vi "monitor fpga rm window status and set dynamic button state.vi"(8 "error in (no error)":errorcluster) -> (0 "error out":errorcluster)   [LabVIEW 2016, in "FPGA RM System Definition API.lvlib"]
uses:
  FPGA RM System Definition API.lvlib
  <vilib>/NI VeriStand/Custom Device API/Custom Device API.lvlib
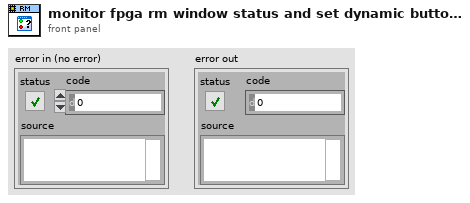
[diagram p1: front panel]
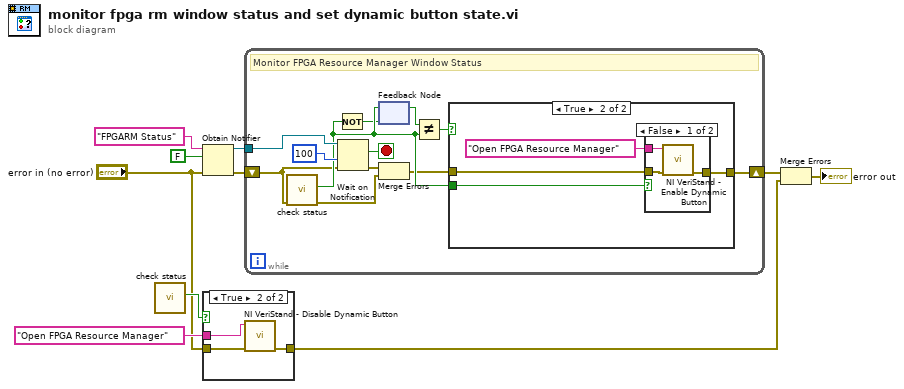
[diagram p0: block diagram]
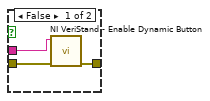
[diagram p2: hidden frame]
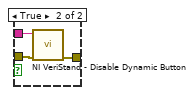
[diagram p4: hidden frame]
diagram:
  n1 = call "check status.vi"() -> ("status"=w6:bool)  [unwired: 10 in, 1 out]
  n2 = Obtain Notifier(name (unnamed)="FPGARM Status", notification data type=FALSE, error in (no error)="error in (no error)") -> (notifier out=w8:refnum<notifier>, error out=w4:errorcluster)  [unwired: 1 in, 1 out]
  n3 = case shown="True" w6 {
    tunnel: "Open FPGA Resource Manager" ("Button ID") -> [w13 w16]
    tunnel: "error in (no error)" -> [w12 w15]
    tunnel: [w11 w14] -> w2
    frame False {
      n4 = call <vilib>:"NI VeriStand - Enable Dynamic Button.vi"("error in (no error)"=w12, "Button ID"=w13) -> ("error out"=w11:errorcluster)  [unwired: 9 in]
    }
    frame True {
      n5 = call <vilib>:"NI VeriStand - Disable Dynamic Button.vi"("error in (no error)"=w15, "Button ID"=w16) -> ("error out"=w14:errorcluster)  [unwired: 9 in]
    }
  }
  n6 = while {
    tunnel: w8 -> [w28]
    shift-right: [w17] -> w3
    shift-left: w4 -> [w21]
    stop <- w27 stop-if-true
    # "Monitor FPGA Resource Manager Window Status"
    n7 = call "check status.vi"("error in (no error)"=w21) -> ("error out"=w19:errorcluster, "status"=w23:bool)  [unwired: 9 in]
    n8 = Not(x=w23) -> (.not. x?=w22:bool)
    n9 = Wait on Notification(notifier=w28, timeout in ms (-1)=100, error in (no error)=w21) -> (notification=w27:bool, error out=w20:errorcluster)  [unwired: 1 in, 2 out]
    n10 = feedback-in #1(w23) -> ()
    n11 = feedback #1(w22) -> (w25:bool)
    n12 = Merge Errors(w20, w19) -> (w18:errorcluster)
    n13 = Not Equal?(x=w25, y=w23) -> (x != y?=w24:bool)
    n14 = case shown="True" w24 {
      tunnel: w23 -> [_ w32]
      tunnel: w18 -> [w29 w31]
      tunnel: [w29 w30] -> w17
      frame False {
      }
      frame True {
        n15 = case shown="False" w32 {
          tunnel: "Open FPGA Resource Manager" ("Button ID") -> [w36 w39]
          tunnel: w31 -> [w35 w38]
          tunnel: [w34 w37] -> w30
          frame False {
            n16 = call <vilib>:"NI VeriStand - Enable Dynamic Button.vi"("error in (no error)"=w35, "Button ID"=w36) -> ("error out"=w34:errorcluster)  [unwired: 9 in]
          }
          frame True {
            n17 = call <vilib>:"NI VeriStand - Disable Dynamic Button.vi"("error in (no error)"=w38, "Button ID"=w39) -> ("error out"=w37:errorcluster)  [unwired: 9 in]
          }
        }
      }
    }
  }
  n18 = Merge Errors(w3, w2) -> (→"error out":errorcluster)
